vi "FTW-CodeGen-AdaptToInputs.vi"(0 "State In":T1, 5 "XRef":refnum<vi>, 7 "Term Types":cluster{"Type":variant, "ID":string}[](array[cluster])) -> (4 "State Out":T1, 6 "Reply":string[](array[string]))   [LabVIEW 2015, in "FTW-SQLite-Insert.xnode"]
uses:
  FTW-SQLite-Insert.xnode
  FTW-CodeGen-State.ctl
  FTW-CodeGen-XNodeReplyType.ctl
panel:
  # "Inputs"
  # "Outputs"
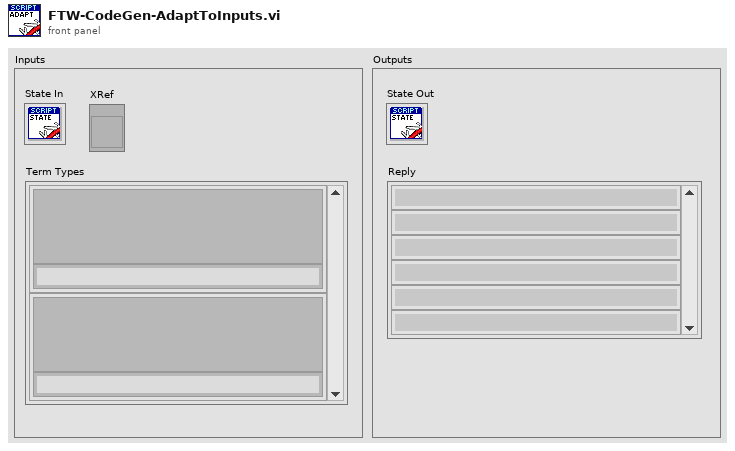
[diagram p1: front panel]
types:
  T1 = typedef "FTW-SQLite-Insert.xnode/FTW-CodeGen-State.ctl" = cluster{"Dummy":i32}
  T2 = typedef "FTW-CodeGen-XNodeReplyType.ctl" = enum16{"UpdateState", "AdaptToInputs", "AdaptAndAugment", "CosmeticUpdate", "NoReply"}
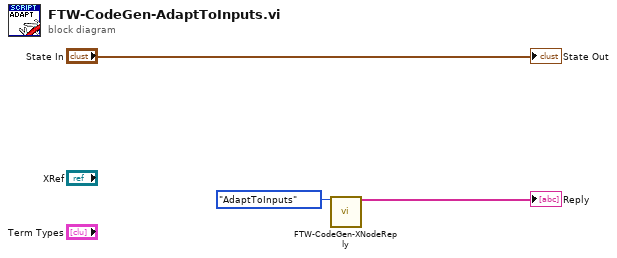
[diagram p0: block diagram]
diagram:
  n1 = call "FTW-CodeGen-XNodeReply.vi"("XNode Reply Type"=FTW-CodeGen-XNodeReplyType."AdaptToInputs") -> ("Reply"=→"Reply":string[])  [unwired: 14 in]
  "State Out" <- "State In"
